vi "Init Callback User Events.vi"(8 "error in":errorcluster, 11 "MyEventGrid in":refnum<class "MyEventGrid.lvclass">) -> (0 "error out":errorcluster, 3 "MyEventGrid out":refnum<class "MyEventGrid.lvclass">)   [LabVIEW 2024, in "MyEventGrid.lvclass"]
uses:
  MyEventGrid.lvclass
  MyEventGrid.lvclass/MyEventGrid.ctl
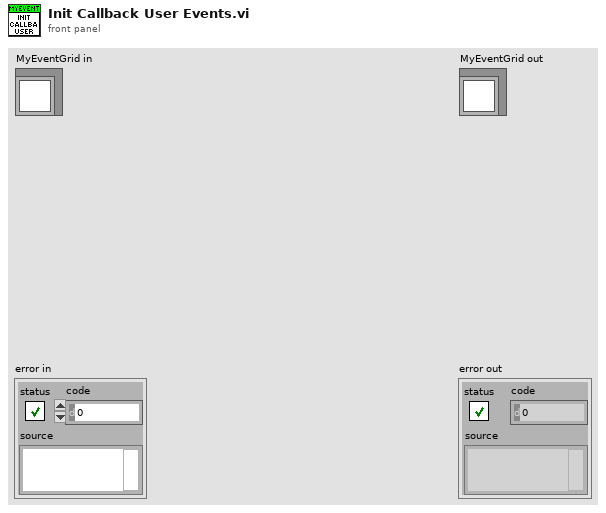
[diagram p1: front panel]
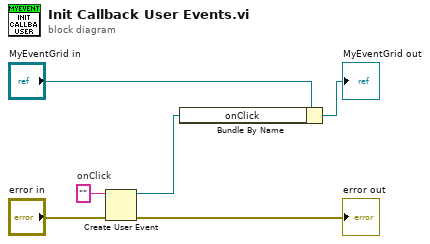
[diagram p0: block diagram]
diagram:
  w6 = ""  # onClick
  n1 = Create User Event(user event datatype=w6, error in="error in") -> (user event=w2:refnum<user-event>, error out=→"error out":errorcluster)
  n2 = Bundle By Name(cluster="MyEventGrid in", "onClick"=w2) -> (→"MyEventGrid out":refnum<class "MyEventGrid.lvclass">)
